vi "Test_Baseline_Jitter.vi"(8 "error in (no error)":errorcluster, 11 "Falttened Array in":string[](array[string])) -> (0 "error out":errorcluster, 1 "Results":T3(array[cluster]), 2 "Pass":bool, 3 "Falttened Array Out":string[](array[string]))   [LabVIEW 2014]
doc: "This example uses an assembly-level call to obtain precise timestamps from RT targets. The purpose of this example is to gather timing information on a user's VI by running it for several iterations. The example obtains several consecutive 64-bit timestamps, which are stored in an array and used later to produce a histogram of execution time. This VI can self-calibrate by subtracting out the overhead of calling NI Get Timestamp.vi from the array of timing data.\n\nINSTRUCTIONS:\n1. Select a number of iterations and warmup iterations to exclude from the benchmark.\n2. Use calibration if you want to exclude the overhead of the timestamping operation.\n3. Go to the diagram and insert the code you want to benchmark."
uses:
  CommonSubVIs/Framework/Flattened_Array/Set Parameter Value by Name (I32).vi
  CommonSubVIs/Framework/Flattened_Array/Set Parameter Value by Name (Double).vi
  CommonSubVIs/Framework/Flattened_Array/Set Parameter Value by Name (Bool).vi
  CommonSubVIs/Framework/Flattened_Array/Get Parameter Value by Name (Bool).vi
  CommonSubVIs/Framework/Flattened_Array/Get Parameter Value by Name I32.vi
  CommonSubVIs/Framework/Flattened_Array/Get Parameter Value by Name (U32).vi
panel:
  in  "stop":bool
  out "Tab Control":enum32{"Jitter", "Other"}(tab)
  out "CPU Cache":bool=TRUE
  out "Loop Iterations":i32=1000
  out "Warmup iterations":i32=50
  out "Desired Repetitions":u32=25
  out "Loop Period (us)":u32=37
  out "Execution Histogram":T1(graph)
  out "Execution Times":dbl[](graph)
  out "Standard deviation (us)":dbl format="%.2f"
  out "Max Jitter (uS)":dbl format="%.2f"
  out "Mean Time (uS)":dbl format="%.2f"
  out "Waveform Chart":T2(graph)
  out "Iterations":i32(slide) caption="Stable Repetitions" min=0 max=100 step=1 scale=0.0..25.0
  out "Maximum Std Dev (us)":dbl
  out "Maximum Jitter (us)":dbl
  # "Settings"
  # "Results for Lastest Repetition"
  # "Overall Test Results"
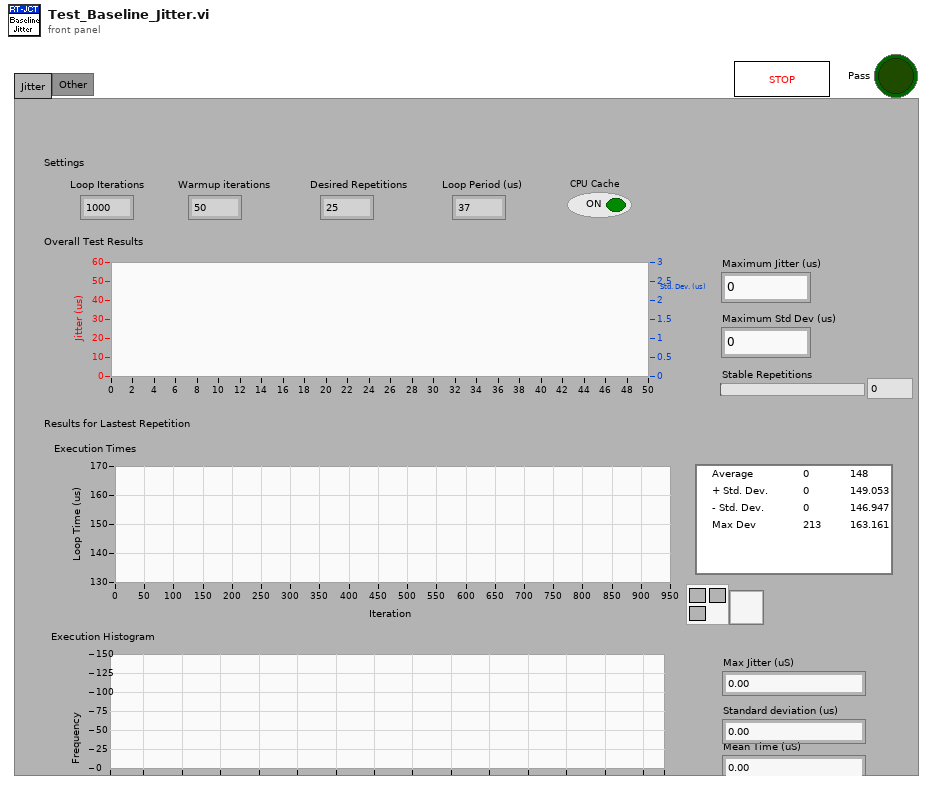
[diagram p1: front panel]
types:
  T1 = cluster{"X Values":dbl[], "Histogram: h(x)":i32[]}
  T2 = cluster{"max jitter (uS)":dbl, "Max Jitter (us)":dbl, "standard deviation (uS)":dbl, "Max Std Dev (us)":dbl}
  T3 = cluster{"Name":string, "Value":dbl, "Units":string, "Format String":string}[]
  T4 = cluster{"Name":string, "Color":u32, "Style":u8, "Point Style":u8, "Name Visible":bool, "Allow Drag":bool, "Cursor Mode":u32, "Plot":i32, "Index":i32, "Position":cluster{"X":dbl, "Y":dbl}, "X Scale":u32, "Y Scale":u32, "Watch Plots":i32[], "Watch All Plots":bool, "Plot Area":i32, "Label Offset":cluster{"X":dbl, "Y":dbl}}[]
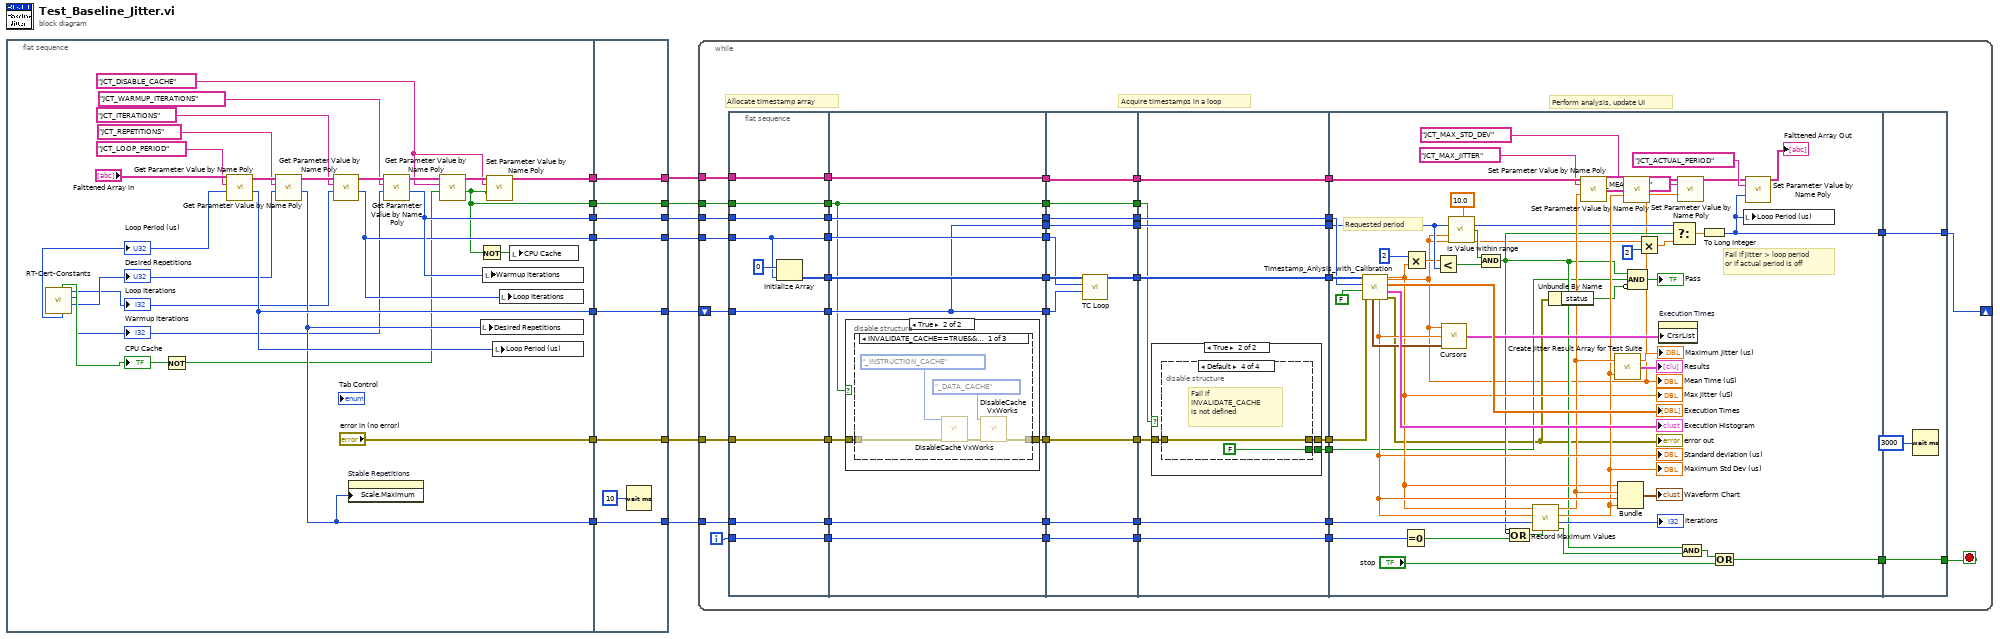
[diagram p0: block diagram]
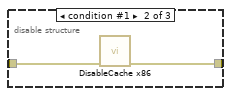
[diagram p3: hidden frame]
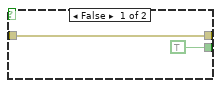
[diagram p5: hidden frame]
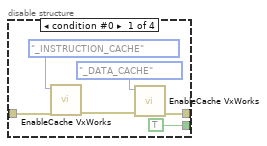
[diagram p6: hidden frame]
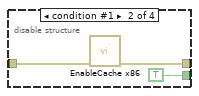
[diagram p7: hidden frame]
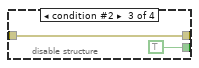
[diagram p8: hidden frame]
diagram:
  n1 = flat-sequence {
    tunnel: [w29] -> w12
    tunnel: ["error in (no error)"] -> w11
    tunnel: [w30] -> w9
    tunnel: [w27] -> w7
    tunnel: [w28] -> w5
    tunnel: [w24] -> w3
    tunnel: [w21] -> w1
    tunnel: [w46] -> w13
    tunnel: [w47] -> w14
    tunnel: w12 -> [w47]
    tunnel: w11 -> [w46]
    tunnel: [w44] -> w10
    tunnel: w9 -> [w44]
    tunnel: [w43] -> w8
    tunnel: w7 -> [w43]
    tunnel: [w42] -> w6
    tunnel: w5 -> [w42]
    tunnel: [w41] -> w4
    tunnel: w3 -> [w41]
    tunnel: [w40] -> w2
    tunnel: w1 -> [w40]
    frame #0 {
      w23 = "JCT_DISABLE_CACHE"
      n2 = call "RT-Cert-Constants.vi"() -> ("Desired Repetitions"=w18:u32, "Warmup Iterations"=w15:i32, "Iterations"=w16:i32, "Loop Period (us)"=w17:u32, "CPU Cache"=w19:bool)  [unwired: 7 in]
      "Desired Repetitions" <- w18
      "Loop Period (us)" <- w17
      "Loop Iterations" <- w16
      "Warmup iterations" <- w15
      "CPU Cache" <- w19
      n3 = Not(x=w19) -> (.not. x?=w22:bool)
      n4 = call-poly "Get Parameter Value by Name Poly.vi"("Default Value"=w17, "Parameter"="JCT_LOOP_PERIOD", "Parameter Array in"="Falttened Array in") -> ("Value"=w30:u32, "Parameter Array Out"=w37:string[])  [unwired: 5 in, 1 out]
      n5 = call-poly "Get Parameter Value by Name Poly.vi"("Default Value"=w18, "Parameter"="JCT_REPETITIONS", "Parameter Array in"=w37) -> ("Value"=w29:u32, "Parameter Array Out"=w36:string[])  [unwired: 5 in, 1 out]
      n6 = call-poly "Get Parameter Value by Name Poly.vi"("Default Value"=w16, "Parameter"="JCT_ITERATIONS", "Parameter Array in"=w36) -> ("Value"=w27:i32, "Parameter Array Out"=w35:string[])  [unwired: 5 in, 1 out]
      n7 = property on="Stable Repetitions" class="Slide (strict)"("Scale.Maximum"=w29) -> ()  [unwired: 2 in, 2 out]
      n8 = call-poly "Get Parameter Value by Name Poly.vi"("Default Value"=w15, "Parameter"="JCT_WARMUP_ITERATIONS", "Parameter Array in"=w35) -> ("Value"=w28:i32, "Parameter Array Out"=w26:string[])  [unwired: 5 in, 1 out]
      n9 = call-poly "Get Parameter Value by Name Poly.vi"("Default Value"=w22, "Parameter"=w23, "Parameter Array in"=w26) -> ("Value"=w21:bool, "Parameter Array Out"=w25:string[])  [unwired: 5 in, 1 out]
      n10 = Not(x=w21) -> (.not. x?=w20:bool)
      n11 = local write "Desired Repetitions"(w29) -> ()
      n12 = local write "Warmup iterations"(w28) -> ()
      n13 = call-poly "Set Parameter Value by Name Poly.vi"("Parameter Array"=w25, "Parameter Name"=w23, "Bool"=w21) -> ("Parameter Array Out"=w24:string[])  [unwired: 9 in, 3 out]
      n14 = local write "Loop Period (us)"(w30) -> ()
      n15 = local write "Loop Iterations"(w27) -> ()
      n16 = local write "CPU Cache"(w20) -> ()
    }
    frame #1 {
      n17 = Wait (ms)(milliseconds to wait=u32 10) -> ()  [unwired: 1 out]
    }
  }
  n18 = while {
    tunnel: w14 -> [w94]
    tunnel: w13 -> [w81]
    tunnel: w8 -> [w76]
    tunnel: w6 -> [w72]
    tunnel: w4 -> [w68]
    tunnel: w2 -> [w64]
    shift-right: [w52] -> _
    shift-left: w10 -> [w77]
    i -> [w93]
    stop <- w50 stop-if-true
    # "Perform analysis, update UI"
    # "Acquire timestamps in a loop"
    # "Allocate timestamp array"
    n19 = flat-sequence {
      tunnel: [w98] -> w92
      tunnel: [w104] -> w91
      tunnel: [w102] -> w90
      tunnel: w94 -> [w102]
      tunnel: [w101] -> w89
      tunnel: w93 -> [w101]
      tunnel: [w100] -> w82
      tunnel: w81 -> [w100]
      tunnel: [w99] -> w78
      tunnel: w77 -> [w99]
      tunnel: w76 -> [w98]
      tunnel: [w97] -> w73
      tunnel: w72 -> [w97]
      tunnel: [w96] -> w69
      tunnel: w68 -> [w96]
      tunnel: [w95] -> w65
      tunnel: w64 -> [w95]
      tunnel: w92 -> [w114]
      tunnel: [w114] -> w62
      tunnel: w91 -> [w113]
      tunnel: [w113] -> w61
      tunnel: w90 -> [w112]
      tunnel: [w112] -> w60
      tunnel: w89 -> [w111]
      tunnel: [w111] -> w59
      tunnel: w82 -> [w110]
      tunnel: [w109] -> w58
      tunnel: [w107] -> w57
      tunnel: w78 -> [w107]
      tunnel: [w108] -> w56
      tunnel: w73 -> [w108]
      tunnel: [w107] -> w55
      tunnel: [w106] -> w54
      tunnel: w69 -> [w106]
      tunnel: [w105] -> w53
      tunnel: w65 -> [w105]
      tunnel: [w129] -> w88
      tunnel: w62 -> [w128]
      tunnel: w61 -> [w130]
      tunnel: [w136] -> w86
      tunnel: w60 -> [w136]
      tunnel: [w135] -> w84
      tunnel: w59 -> [w135]
      tunnel: w58 -> [w134]
      tunnel: [w134] -> w80
      tunnel: w57 -> [w127]
      tunnel: [w133] -> w74
      tunnel: w56 -> [w133]
      tunnel: w55 -> [w132]
      tunnel: [w132] -> w70
      tunnel: w54 -> [w131]
      tunnel: [w131] -> w66
      tunnel: w53 -> [w126]
      tunnel: [w126] -> w63
      tunnel: w88 -> [w146]
      tunnel: [w146] -> w87
      tunnel: w86 -> [w145]
      tunnel: [w145] -> w85
      tunnel: w84 -> [w144]
      tunnel: [w144] -> w83
      tunnel: w80 -> [w143]
      tunnel: [w142] -> w79
      tunnel: [w141] -> w75
      tunnel: w74 -> [w141]
      tunnel: [w140] -> w71
      tunnel: w70 -> [w140]
      tunnel: [w139] -> w67
      tunnel: w66 -> [w139]
      tunnel: w63 -> [w138]
      tunnel: [w137] -> w48
      tunnel: w87 -> [w212]
      tunnel: w85 -> [w203]
      tunnel: w83 -> [w202]
      tunnel: w79 -> [w200]
      tunnel: w75 -> [w199]
      tunnel: w71 -> [w183]
      tunnel: w67 -> [w198]
      tunnel: [w178] -> w51
      tunnel: [w180] -> w49
      tunnel: w48 -> [w172]
      tunnel: [w214] -> w52
      tunnel: w51 -> [w214]
      tunnel: [w213] -> w50
      tunnel: w49 -> [w213]
      frame #0 {
        n20 = Initialize Array(u64 0, w98) -> (w104:u64[])
      }
      frame #1 {
        n21 = case shown="True" w105 {
          tunnel: w110 -> [w115 w117]
          tunnel: [w115 w116] -> w109
          frame False {
          }
          frame True {
            n22 = disable-structure shown="INVALIDATE_CACHE==TRUE&&OS==VxWorks" {
              disable-tunnel: w117 -> [w122 w124 w125]
              disable-tunnel: [w120 w123 w125] -> w116
              frame condition #0 {
                n23 = call "DisableCache VxWorks.vi"("error in (no error)"=w122, "Cache Type"=enum16{"_INSTRUCTION_CACHE", "_DATA_CACHE"}."_INSTRUCTION_CACHE") -> ("error out"=w121:errorcluster)  [unwired: 8 in, 1 out]
                n24 = call "DisableCache VxWorks.vi"("error in (no error)"=w121, "Cache Type"=enum16{"_INSTRUCTION_CACHE", "_DATA_CACHE"}."_DATA_CACHE") -> ("error out"=w120:errorcluster)  [unwired: 8 in, 1 out]
              }
              frame condition #1 {
                n25 = call "DisableCache x86.vi"("error in (no error)"=w124) -> ("error out"=w123:errorcluster)  [unwired: 10 in]
              }
              frame condition #2 (active) {
              }
            }
          }
        }
      }
      frame #2 {
        n26 = call "TC Loop.vi"("Period (us)"=w127, "Iterations"=w128, "Pre-allocated Timestamp Array"=w130) -> ("Timestamp Array"=w129:u64[])  [unwired: 8 in]
      }
      frame #3 {
        n27 = case shown="True" w138 {
          tunnel: w143 -> [w148 w151]
          tunnel: [w148 w150] -> w142
          tunnel: [TRUE w149] -> w137
          frame False {
          }
          frame True {
            n28 = disable-structure shown="Default" {
              disable-tunnel: w151 -> [w157 w160 w162 w164]
              disable-tunnel: [w156 w159 w162 w164] -> w150
              disable-tunnel: [TRUE TRUE TRUE FALSE] -> w149
              frame condition #0 {
                n29 = call "EnableCache VxWorks.vi"("error in (no error)"=w157, "Cache Type"=enum16{"_INSTRUCTION_CACHE", "_DATA_CACHE"}."_INSTRUCTION_CACHE") -> ("error out"=w155:errorcluster)  [unwired: 8 in, 1 out]
                n30 = call "EnableCache VxWorks.vi"("error in (no error)"=w155, "Cache Type"=enum16{"_INSTRUCTION_CACHE", "_DATA_CACHE"}."_DATA_CACHE") -> ("error out"=w156:errorcluster)  [unwired: 8 in, 1 out]
              }
              frame condition #1 {
                n31 = call "EnableCache x86.vi"("error in (no error)"=w160) -> ("error out"=w159:errorcluster)  [unwired: 10 in]
              }
              frame condition #2 {
              }
              frame condition #3 (active) {
                # "Fail if\nINVALIDATE_CACHE\nis not defined"
              }
            }
          }
        }
      }
      frame #4 {
        # "Fail if jitter > loop period\nor if actual period is off"
        # "Requested period"
        n32 = call "Timestamp_Anlysis_with_Calibration.vi"("error in (no error)"=w200, "Calibrate?"=FALSE, "Warmup iterations"=w199, "Timestamp Array"=w212) -> ("error out"=w170:errorcluster, "execution histogram"=→"Execution Histogram":T1, "execution times (uS)"=→"Execution Times":dbl[], "max jitter (uS)"=w175:dbl, "standard deviation (uS)"=w201:dbl, "mean time (uS)"=w165:dbl, "Max Jitter Point"=w206:cluster{"X":dbl, "Y":dbl})  [unwired: 1 in]
        "Max Jitter (uS)" <- w175
        "Standard deviation (us)" <- w201
        "Mean Time (uS)" <- w165
        "error out" <- w170
        n33 = Equal To 0?(x=w202) -> (x = 0?=w182:bool)
        n34 = Multiply(x=u32 2 ("y"), y=w175) -> (x*y=w174:dbl)
        n35 = Less?(x=w174, y=w183) -> (x < y?=w187:bool)
        n36 = call "Cursors.vi"("Max Jitter Point"=w206, "standard deviation"=w201, "mean"=w165) -> ("Cursor List"=w208:T4)
        n37 = call "Is Value within range.vi"("%"=10.0, "Target"=w183, "Value"=w165) -> ("In Range?"=w188:bool)  [unwired: 10 in, 2 out]
        n38 = Compound Arithmetic op=AND(w188, w187) -> (w173:bool)
        n39 = Compound Arithmetic op=OR(invert w173, w182) -> (w181:bool)
        n40 = call "Record Maximum Values.vi"("Reset"=w181, "Desired Iterations"=w203, "standard deviation (us)"=w201, "jitter (us)"=w175) -> ("Stable?"=w184:bool, "Stable Iterations"=→"Iterations":i32, "Max Std Dev (us)"=w194:dbl, "Max Jitter (us)"=w196:dbl)  [unwired: 3 in]
        "Maximum Std Dev (us)" <- w194
        "Maximum Jitter (us)" <- w196
        n41 = Unbundle By Name(w170) -> ("status"=w169:bool)
        n42 = call-poly "Set Parameter Value by Name Poly.vi"("Parameter Array"=w198, "Parameter Name"="JCT_MAX_JITTER", "Double"=w196) -> ("Parameter Array Out"=w195:string[])  [unwired: 9 in, 3 out]
        n43 = call "Create Jitter Result Array for Test Suite.vi"("standard deviation (uS)"=w194, "max jitter (uS)"=w196) -> ("Results"=→"Results":T3)
        n44 = Bundle("max jitter (uS)"=w175, "Max Jitter (us)"=w196, "standard deviation (uS)"=w201, "Max Std Dev (us)"=w194) -> (→"Waveform Chart":T2)  [unwired: 1 in]
        n45 = call-poly "Set Parameter Value by Name Poly.vi"("Parameter Array"=w195, "Parameter Name"="JCT_MAX_STD_DEV", "Double"=w194) -> ("Parameter Array Out"=w168:string[])  [unwired: 9 in, 3 out]
        n46 = Compound Arithmetic op=AND(w173, w172, invert w169) -> (→"Pass":bool)
        n47 = Multiply(x=w165, y=u32 2) -> (x*y=w190:dbl)
        n48 = property on="Execution Times" class="WFGraph (strict)"("CrsrList"=w208) -> ()  [unwired: 2 in, 2 out]
        n49 = Select(t=w183, s=w173, f=w190) -> (s? t:f=w189:dbl)
        n50 = call-poly "Set Parameter Value by Name Poly.vi"("Parameter Array"=w168, "Parameter Name"="JCT_MEAN_TIME", "Double"=w165) -> ("Parameter Array Out"=w167:string[])  [unwired: 9 in, 3 out]
        n51 = And(x=w173, y=w184) -> (x .and. y?=w186:bool)
        n52 = To Long Integer(number=w189) -> (32bit integer=w178:i32)
        n53 = Or(x=w186, y="stop") -> (x .or. y?=w180:bool)
        n54 = local write "Loop Period (us)"(w178) -> ()
        n55 = call-poly "Set Parameter Value by Name Poly.vi"("Parameter Array"=w167, "Parameter Name"="JCT_ACTUAL_PERIOD", "I32"=w178) -> ("Parameter Array Out"=→"Falttened Array Out":string[])  [unwired: 9 in, 3 out]
      }
      frame #5 {
        n56 = Wait (ms)(milliseconds to wait=u32 3000) -> ()  [unwired: 1 out]
      }
    }
  }
